vi "SM Ref Taversal Callback.vi"(8 "error in (no error)":errorcluster, 9 "GObj Refnum":refnum<vi>, 11 "Refs In":T1) -> (0 "error out":errorcluster, 1 "Stop Traversal?":bool, 3 "Refs":T1)   [LabVIEW 2022 SP3, in "FlexBlocks Support.lvlib"]
uses:
  FlexBlocks Support.lvlib
  SM Refs.ctl
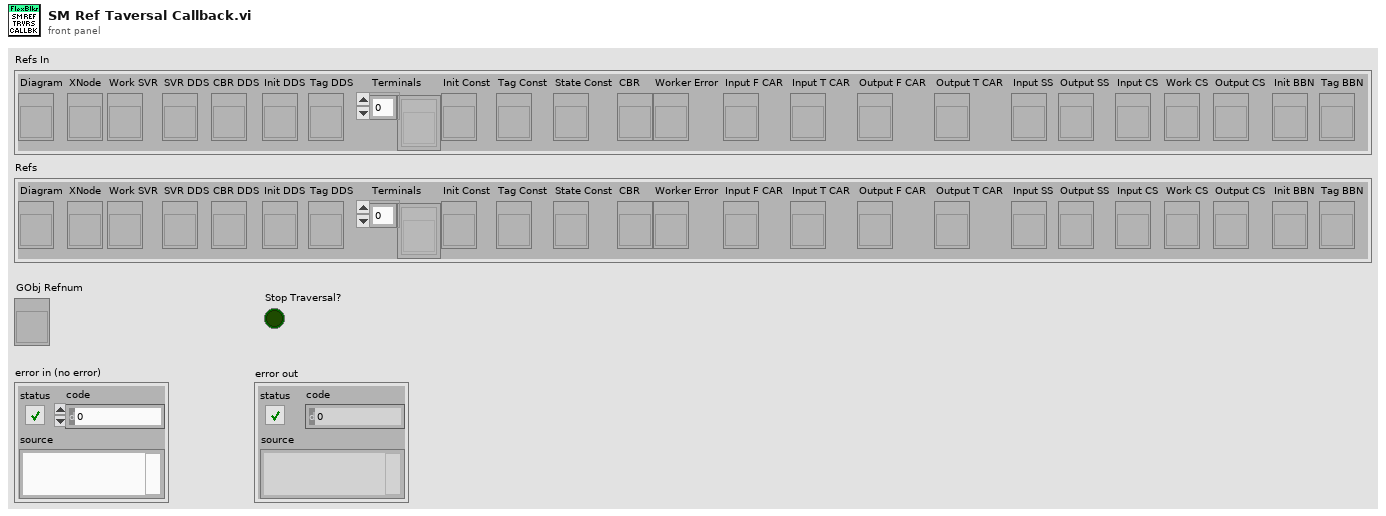
[diagram p1: front panel]
types:
  T1 = typedef "FlexBlocks Support.lvlib/SM Refs.ctl" = cluster{"Diagram":refnum<vi>, "XNode":refnum<vi>, "Work SVR":refnum<vi>, "SVR DDS":refnum<vi>, "CBR DDS":refnum<vi>, "Init DDS":refnum<vi>, "Tag DDS":refnum<vi>, "Terminals":refnum<vi>[], "Init Const":refnum<vi>, "Tag Const":refnum<vi>, "State Const":refnum<vi>, "CBR":refnum<vi>, "Worker Error":refnum<vi>, "Input F CAR":refnum<vi>, "Input T CAR":refnum<vi>, "Output F CAR":refnum<vi>, "Output T CAR":refnum<vi>, "Input SS":refnum<vi>, "Output SS":refnum<vi>, "Input CS":refnum<vi>, "Work CS":refnum<vi>, "Output CS":refnum<vi>, "Init BBN":refnum<vi>, "Tag BBN":refnum<vi>}
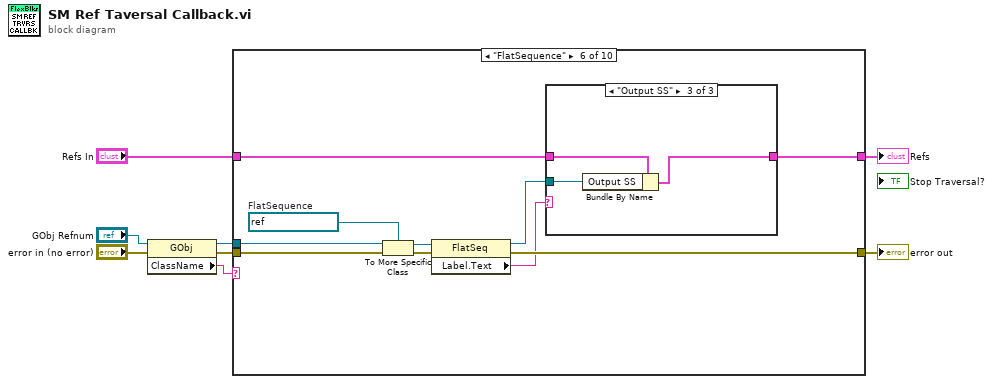
[diagram p0: block diagram]
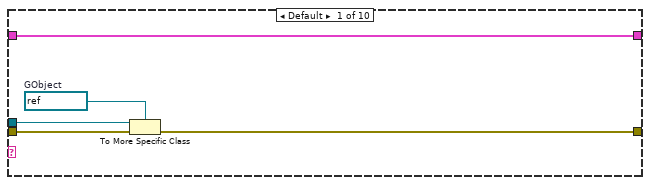
[diagram p2: hidden frame]
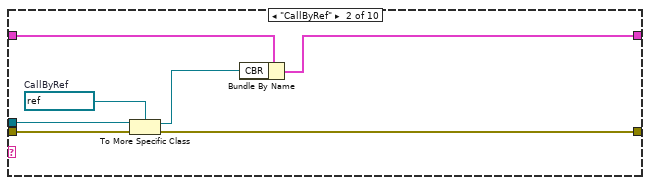
[diagram p3: hidden frame]
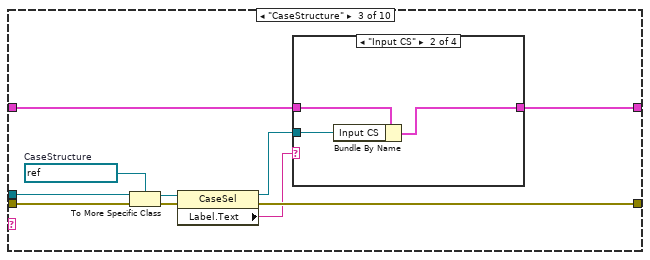
[diagram p4: hidden frame]
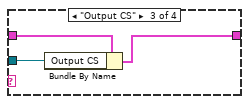
[diagram p6: hidden frame]
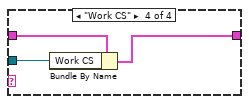
[diagram p7: hidden frame]
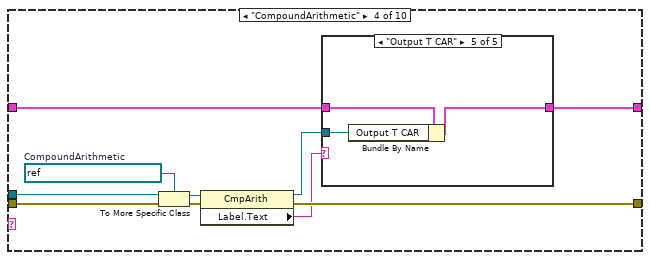
[diagram p8: hidden frame]
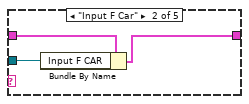
[diagram p10: hidden frame]
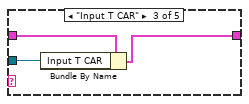
[diagram p11: hidden frame]
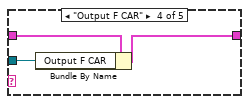
[diagram p12: hidden frame]
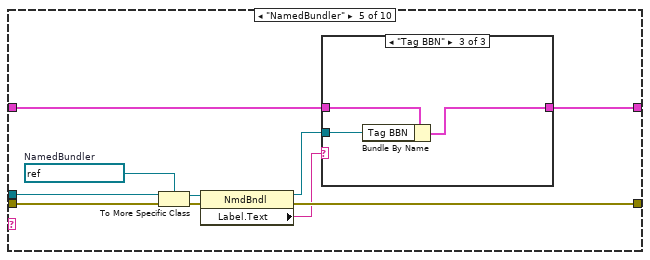
[diagram p13: hidden frame]
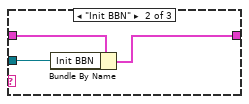
[diagram p15: hidden frame]
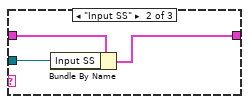
[diagram p17: hidden frame]
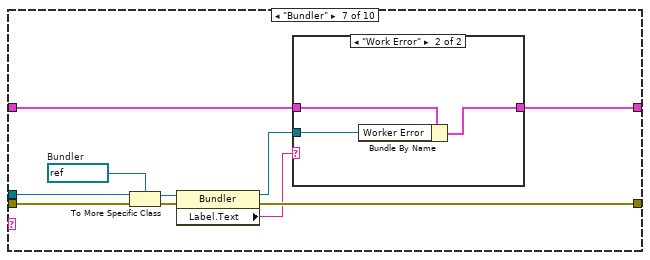
[diagram p18: hidden frame]
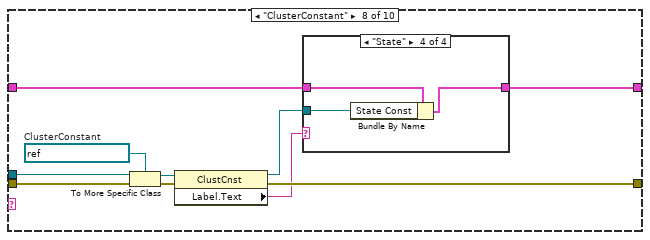
[diagram p20: hidden frame]
diagram:
  n1 = property class="GObj"(reference="GObj Refnum", error in="error in (no error)") -> (reference out=w6:refnum<vi>, error out=w4:errorcluster, "ClassName"=w7:string)
  n2 = case shown="\"FlatSequence\"" w7 {
    tunnel: w6 -> [w11 w19 w29 w49 w72 w89 w106 w120 w138 w147]
    tunnel: w4 -> [w12 w20 w30 w50 w73 w90 w107 w121 w137 w148]
    tunnel: "Refs In" -> [w13 w14 w22 w42 w65 w82 w99 w115 w132 w141]
    tunnel: [w13 w15 w21 w41 w64 w81 w98 w112 w133 w139] -> w2
    tunnel: [w9 w17 w26 w46 w69 w86 w103 w117 w134 w140] -> w1
    frame Default {
      w10 = refnum<vi> refnum  # GObject
      n3 = To More Specific Class(target class=w10, reference=w11, error in=w12) -> (error out=w9:errorcluster)  [unwired: 1 out]
    }
    frame "CallByRef" {
      w18 = refnum<vi> refnum  # CallByRef
      n4 = To More Specific Class(target class=w18, reference=w19, error in=w20) -> (specific class reference=w16:refnum<vi>, error out=w17:errorcluster)
      n5 = Bundle By Name(cluster=w14, "CBR"=w16) -> (w15:T1)
    }
    frame "CaseStructure" {
      w28 = refnum<vi> refnum  # CaseStructure
      n6 = To More Specific Class(target class=w28, reference=w29, error in=w30) -> (specific class reference=w25:refnum<vi>, error out=w27:errorcluster)
      n7 = property class="CaseSel"(reference=w25, error in=w27) -> (reference out=w24:refnum<vi>, error out=w26:errorcluster, "Label.Text"=w23:string)
      n8 = case shown="\"Input CS\"" w23 {
        tunnel: w24 -> [_ w33 w36 w39]
        tunnel: w22 -> [w31 w34 w37 w40]
        tunnel: [w31 w32 w35 w38] -> w21
        frame Default {
        }
        frame "Input CS" {
          n9 = Bundle By Name(cluster=w34, "Input CS"=w33) -> (w32:T1)
        }
        frame "Output CS" {
          n10 = Bundle By Name(cluster=w37, "Output CS"=w36) -> (w35:T1)
        }
        frame "Work CS" {
          n11 = Bundle By Name(cluster=w40, "Work CS"=w39) -> (w38:T1)
        }
      }
    }
    frame "CompoundArithmetic" {
      w48 = refnum<vi> refnum  # CompoundArithmetic
      n12 = To More Specific Class(target class=w48, reference=w49, error in=w50) -> (specific class reference=w45:refnum<vi>, error out=w47:errorcluster)
      n13 = property class="CmpArith"(reference=w45, error in=w47) -> (reference out=w44:refnum<vi>, error out=w46:errorcluster, "Label.Text"=w43:string)
      n14 = case shown="\"Output T CAR\"" w43 {
        tunnel: w44 -> [_ w53 w56 w59 w62]
        tunnel: w42 -> [w51 w54 w57 w60 w63]
        tunnel: [w51 w52 w55 w58 w61] -> w41
        frame Default {
        }
        frame "Input F Car" {
          n15 = Bundle By Name(cluster=w54, "Input F CAR"=w53) -> (w52:T1)
        }
        frame "Input T CAR" {
          n16 = Bundle By Name(cluster=w57, "Input T CAR"=w56) -> (w55:T1)
        }
        frame "Output F CAR" {
          n17 = Bundle By Name(cluster=w60, "Output F CAR"=w59) -> (w58:T1)
        }
        frame "Output T CAR" {
          n18 = Bundle By Name(cluster=w63, "Output T CAR"=w62) -> (w61:T1)
        }
      }
    }
    frame "NamedBundler" {
      w71 = refnum<vi> refnum  # NamedBundler
      n19 = To More Specific Class(target class=w71, reference=w72, error in=w73) -> (specific class reference=w68:refnum<vi>, error out=w70:errorcluster)
      n20 = property class="NmdBndl"(reference=w68, error in=w70) -> (reference out=w67:refnum<vi>, error out=w69:errorcluster, "Label.Text"=w66:string)
      n21 = case shown="\"Tag BBN\"" w66 {
        tunnel: w67 -> [_ w76 w79]
        tunnel: w65 -> [w74 w77 w80]
        tunnel: [w74 w75 w78] -> w64
        frame Default {
        }
        frame "Init BBN" {
          n22 = Bundle By Name(cluster=w77, "Init BBN"=w76) -> (w75:T1)
        }
        frame "Tag BBN" {
          n23 = Bundle By Name(cluster=w80, "Tag BBN"=w79) -> (w78:T1)
        }
      }
    }
    frame "FlatSequence" {
      w88 = refnum<vi> refnum  # FlatSequence
      n24 = To More Specific Class(target class=w88, reference=w89, error in=w90) -> (specific class reference=w85:refnum<vi>, error out=w87:errorcluster)
      n25 = property class="FlatSeq"(reference=w85, error in=w87) -> (reference out=w84:refnum<vi>, error out=w86:errorcluster, "Label.Text"=w83:string)
      n26 = case shown="\"Output SS\"" w83 {
        tunnel: w84 -> [_ w93 w96]
        tunnel: w82 -> [w91 w94 w97]
        tunnel: [w91 w92 w95] -> w81
        frame Default {
        }
        frame "Input SS" {
          n27 = Bundle By Name(cluster=w94, "Input SS"=w93) -> (w92:T1)
        }
        frame "Output SS" {
          n28 = Bundle By Name(cluster=w97, "Output SS"=w96) -> (w95:T1)
        }
      }
    }
    frame "Bundler" {
      w105 = refnum<vi> refnum  # Bundler
      n29 = To More Specific Class(target class=w105, reference=w106, error in=w107) -> (specific class reference=w102:refnum<vi>, error out=w104:errorcluster)
      n30 = property class="Bundler"(reference=w102, error in=w104) -> (reference out=w101:refnum<vi>, error out=w103:errorcluster, "Label.Text"=w100:string)
      n31 = case shown="\"Work Error\"" w100 {
        tunnel: w101 -> [_ w110]
        tunnel: w99 -> [w108 w111]
        tunnel: [w108 w109] -> w98
        frame Default {
        }
        frame "Work Error" {
          n32 = Bundle By Name(cluster=w111, "Worker Error"=w110) -> (w109:T1)
        }
      }
    }
    frame "ClusterConstant" {
      w119 = refnum<vi> refnum  # ClusterConstant
      n33 = To More Specific Class(target class=w119, reference=w120, error in=w121) -> (specific class reference=w116:refnum<vi>, error out=w118:errorcluster)
      n34 = property class="ClustCnst"(reference=w116, error in=w118) -> (reference out=w113:refnum<vi>, error out=w117:errorcluster, "Label.Text"=w114:string)
      n35 = case shown="\"State\"" w114 {
        tunnel: w115 -> [w122 w125 w128 w131]
        tunnel: w113 -> [_ w124 w127 w130]
        tunnel: [w122 w123 w126 w129] -> w112
        frame Default {
        }
        frame "Init" {
          n36 = Bundle By Name(cluster=w125, "Init Const"=w124) -> (w123:T1)
        }
        frame "Tag" {
          n37 = Bundle By Name(cluster=w128, "Tag Const"=w127) -> (w126:T1)
        }
        frame "State" {
          n38 = Bundle By Name(cluster=w131, "State Const"=w130) -> (w129:T1)
        }
      }
    }
    frame "StaticVIReference" {
      w136 = refnum<vi> refnum  # StaticVIReference
      n39 = To More Specific Class(target class=w136, reference=w138, error in=w137) -> (specific class reference=w135:refnum<vi>, error out=w134:errorcluster)
      n40 = Bundle By Name(cluster=w132, "Work SVR"=w135) -> (w133:T1)
    }
    frame "DisableStructure" {
      w146 = refnum<vi> refnum  # DisableStructure
      n41 = To More Specific Class(target class=w146, reference=w147, error in=w148) -> (specific class reference=w145:refnum<vi>, error out=w144:errorcluster)
      n42 = property class="DisableStructure"(reference=w145, error in=w144) -> (reference out=w142:refnum<vi>, error out=w140:errorcluster, "Label.Text"=w143:string)
      n43 = case shown="Default" w143 {
        tunnel: w142 -> [_ w151 w154 w157 w160]
        tunnel: w141 -> [w149 w152 w155 w158 w161]
        tunnel: [w149 w150 w153 w156 w159] -> w139
        frame Default {
        }
        frame "SVR DDS" {
          n44 = Bundle By Name(cluster=w152, "SVR DDS"=w151) -> (w150:T1)
        }
        frame "CBR DDS" {
          n45 = Bundle By Name(cluster=w155, "CBR DDS"=w154) -> (w153:T1)
        }
        frame "Init DDS" {
          n46 = Bundle By Name(cluster=w158, "Init DDS"=w157) -> (w156:T1)
        }
        frame "Tag DDS" {
          n47 = Bundle By Name(cluster=w161, "Tag DDS"=w160) -> (w159:T1)
        }
      }
    }
  }
  "Refs" <- w2
  "error out" <- w1
